vi "NI-Digital Loopback and Compare.vi"() -> ()   [LabVIEW 2021]
doc: "Overview\nDemonstrates how to use the NI-Digital Pattern Driver API to create and configure an instrument session and to burst a pattern on the digital pattern instrument, while checking for pass/fail conditions in a loopback configuration."
uses:
  <instrlib>/niDigital/niDigital.llb/niDigital Burst Pattern (Pass Fail).vi
  <instrlib>/niDigital/niDigital.llb/niDigital Selected Function.ctl
panel:
  in  "error in":errorcluster
  out "Square Pass?":bool[](array[boolean])
  in  "Square Wave":refnum<k15>="PXI1Slot2,PXI1Slot3" caption="resource name"
  out "error out":errorcluster
  in  "Simulate?":bool=TRUE
  in  "Sine Wave":refnum<k15>="PXI1Slot2,PXI1Slot3" caption="resource name"
  out "Sine Pass?":bool[](array[boolean])
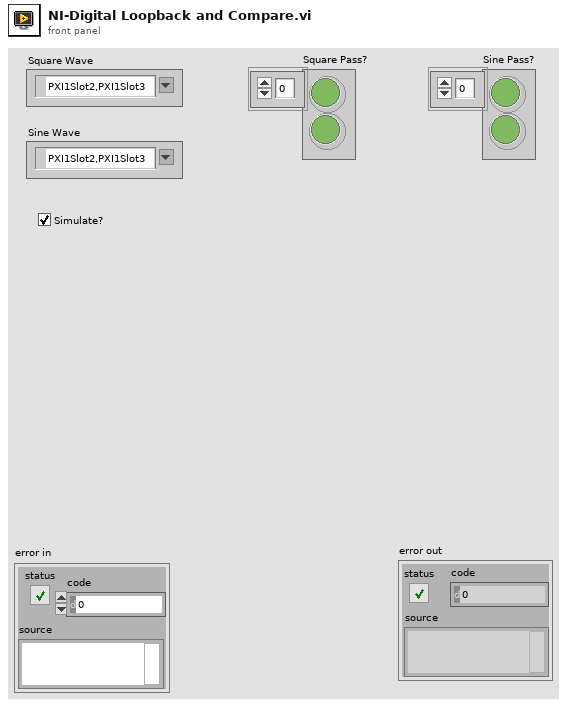
[diagram p1: front panel]
types:
  T1 = typedef "niDigital Selected Function.ctl" = i32
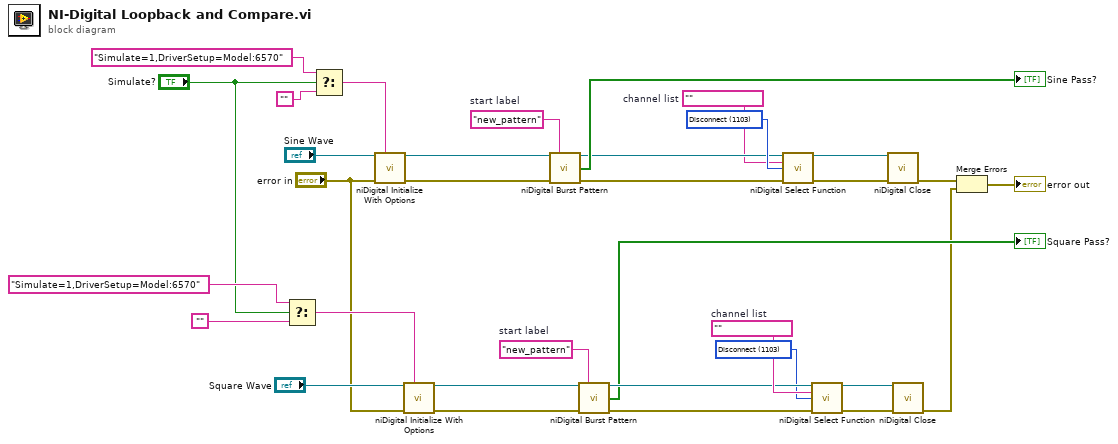
[diagram p0: block diagram]
diagram:
  w9 = T1 1103 items=["Digital"=1100, "PPMU"=1101, "Off"=1102, "Disconnect"=1103] ("function")
  w14 = ""  # channel list
  w5 = "new_pattern"  # start label
  w29 = T1 1103 items=["Digital"=1100, "PPMU"=1101, "Off"=1102, "Disconnect"=1103] ("function")
  w24 = ""  # channel list
  w33 = "new_pattern"  # start label
  n1 = Select(t="Simulate=1,DriverSetup=Model:6570", s="Simulate?", f="") -> (s? t:f=w17:string)
  n2 = Select(t="Simulate=1,DriverSetup=Model:6570", s="Simulate?", f="") -> (s? t:f=w21:string)
  n3 = call <instrlib>:"niDigital Initialize With Options.vi"("resource name"="Sine Wave", "option string"=w21, "error in"="error in") -> ("instrument handle"=w32:refnum<k15>, "error out"=w31:errorcluster)  [unwired: 11 in]
  n4 = call <instrlib>:"niDigital Initialize With Options.vi"("resource name"="Square Wave", "option string"=w17, "error in"="error in") -> ("instrument handle"=w6:refnum<k15>, "error out"=w7:errorcluster)  [unwired: 11 in]
  n5 = call-poly <instrlib>:"niDigital Burst Pattern.vi"("instrument handle"=w32, "start label"=w33, "error in"=w31) -> ("instrument handle out"=w28:refnum<k15>, "pass"=→"Sine Pass?":bool[], "error out"=w27:errorcluster)  [unwired: 10 in]
  n6 = call-poly <instrlib>:"niDigital Burst Pattern.vi"("instrument handle"=w6, "start label"=w5, "error in"=w7) -> ("instrument handle out"=w10:refnum<k15>, "pass"=→"Square Pass?":bool[], "error out"=w11:errorcluster)  [unwired: 10 in]
  n7 = call <instrlib>:"niDigital Select Function.vi"("instrument handle"=w28, "channel list"=w24, "function"=w29, "error in"=w27) -> ("instrument handle out"=w26:refnum<k15>, "error out"=w25:errorcluster)  [unwired: 10 in]
  n8 = call <instrlib>:"niDigital Select Function.vi"("instrument handle"=w10, "channel list"=w14, "function"=w9, "error in"=w11) -> ("instrument handle out"=w12:refnum<k15>, "error out"=w13:errorcluster)  [unwired: 10 in]
  n9 = call <instrlib>:"niDigital Close.vi"("instrument handle"=w26, "error in"=w25) -> ("error out"=w19:errorcluster)  [unwired: 13 in]
  n10 = call <instrlib>:"niDigital Close.vi"("instrument handle"=w12, "error in"=w13) -> ("error out"=w2:errorcluster)  [unwired: 13 in]
  n11 = Merge Errors(w19, w2) -> (→"error out":errorcluster)
